vi "Sequence.Test.Load.Ready.vi"(9 "#products in the machine":i32, 10 "Data in":T9, 11 "Code in":T2={"Ready"=FALSE, "DoubleOrder"=FALSE, "OrderDone"=FALSE, "AllowSingleSlot"=FALSE, "CheckDM"=FALSE, "ThresholdA"=0, "ThresholdB"=0, "Plate"=enum."Wabco", "ImgPath"=path "", "Variant"={"State"=enum."Init", "ImgPath"=path "", "WabcoPlate"="", "WabcoProduct"="", "ClientProduct"="", "ClientPlate"="", "TotalQuantity"=0, "OrderQuantity"=0, "Serial"=0, "Wabco"={"LaserJob"="", "AdditionalTxt"="037", "FactoryCode"="", "RevID"=0, "ForkID"=0, "FailuresLimit"=0, "GlobalCnt"=0, "Bank"=0, "SerialFormat"=enum."6 dig", "CoordA"={"X"=0.0, "Y"=0.0, "Angle"=0.0}, "CoordB"={"X"=0.0, "Y"=0.0, "Angle"=0.0}, "DMCconfig"=0}, "Client"={"LaserJob"="", "AdditionalTxt"="", "FactoryCode"="037", "RevID"=0, "ForkID"=0, "FailuresLimit"=0, "GlobalCnt"=0, "Bank"=0, "SerialFormat"=enum."6 dig", "CoordA"={"X"=0.0, "Y"=0.0, "Angle"=0.0}, "CoordB"={"X"=0.0, "Y"=0.0, "Angle"=0.0}, "DMCconfig"=0}}}) -> (1 "Ready":bool, 2 "Loaded":bool, 3 "StatusFlags":T1)   [LabVIEW 2016]
uses:
  Sequence.Test.Status.ctl
  Sequence.Slot.StatusData.ctl
  Sequence.Test.Unload.Status.ctl
  Sequence.Prod.StatusData.ctl
  Sequence.Step.Status.ctl
  Sequence.Test.BreakReason.ctl
  Sequence.Code.Sets.ctl
  Sequence.PlateType.ctl
  Logger/Logger.Variant.Sets.ctl
  Station/Station.Changeover.State.vi
  Station/Station.Plate.Properties.ctl
  Sequence.Code.SerialFormat.ctl
  Drivers/V7310/LowLevel/V7310.Job.Sets.ctl
  Sequence.SerialsFglb.StatusFlags.ctl
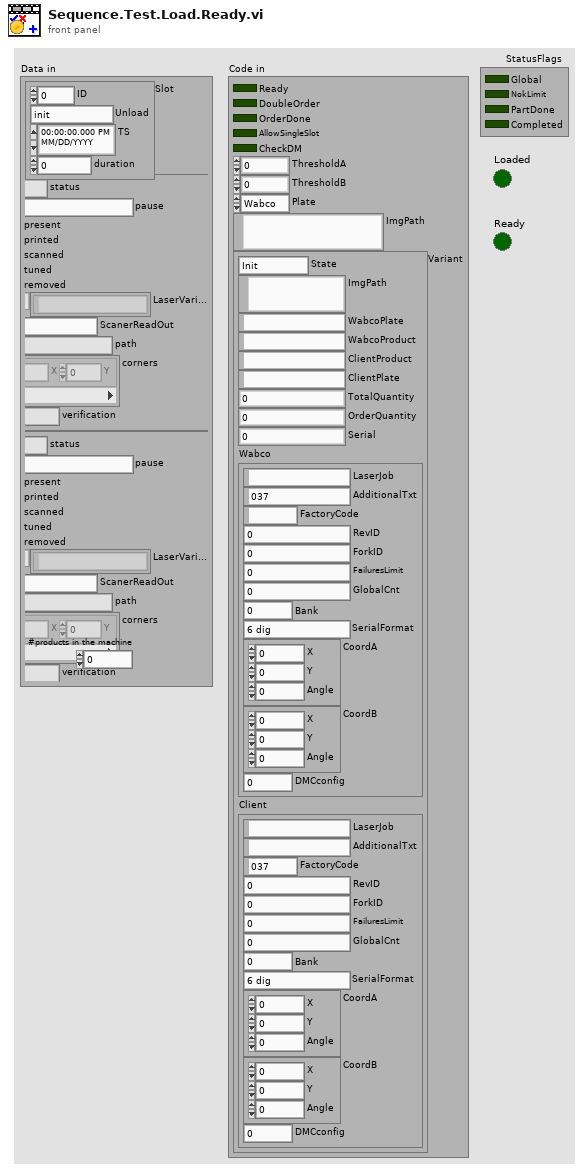
[diagram p1: front panel]
types:
  T1 = typedef "Sequence.SerialsFglb.StatusFlags.ctl" = cluster{"Global":bool, "NokLimit":bool, "PartDone":bool, "Completed":bool}
  T2 = typedef "Sequence.Code.Sets.ctl" = cluster{"Ready":bool, "DoubleOrder":bool, "OrderDone":bool, "AllowSingleSlot":bool, "CheckDM":bool, "ThresholdA":u8, "ThresholdB":u8, "Plate":T3, "ImgPath":path, "Variant":T4}
  T3 = typedef "Sequence.PlateType.ctl" = enum16{"Wabco", "Client"}
  T4 = typedef "Logger.Variant.Sets.ctl" = cluster{"State":T5, "ImgPath":path, "WabcoPlate":string, "WabcoProduct":string, "ClientProduct":string, "ClientPlate":string, "TotalQuantity":u16, "OrderQuantity":u16, "Serial":i32, "Wabco":T6, "Client":T6}
  T5 = typedef "Station.Changeover.State.vi" = enum16{"Init", "Scaning", "NOK", "Wait for ack", "Ready"}
  T6 = typedef "Station.Plate.Properties.ctl" = cluster{"LaserJob":string, "AdditionalTxt":string, "FactoryCode":string, "RevID":u8, "ForkID":u8, "FailuresLimit":u16, "GlobalCnt":i32, "Bank":u8, "SerialFormat":T7, "CoordA":T8, "CoordB":T8, "DMCconfig":i32}
  T7 = typedef "Sequence.Code.SerialFormat.ctl" = enum8{"", "6 dig", "7 dig"}
  T8 = typedef "V7310.Job.Sets.ctl" = cluster{"X":dbl, "Y":dbl, "Angle":dbl}
  T9 = typedef "Sequence.Test.Status.ctl" = cluster{"Slot":T10, "A":T12, "B":T12}
  T10 = typedef "Sequence.Slot.StatusData.ctl" = cluster{"ID":i32, "Unload":T11, "TS":timestamp, "duration":u32}
  T11 = typedef "Sequence.Test.Unload.Status.ctl" = enum16{"init", "check NOK", "check OK", "wait on NOK", "wait on OK", "wait on Unload", "done"}
  T12 = typedef "Sequence.Prod.StatusData.ctl" = cluster{"status":T13, "pause":T14, "present":bool, "printed":bool, "scanned":bool, "tuned":bool, "removed":bool, "LaserVariables":string[], "ScanerReadOut":string, "path":path, "corners":cluster{"X":i32, "Y":i32}[], "verification":u8}
  T13 = typedef "Sequence.Step.Status.ctl" = enum16{"-", "Pending", "Running", "Skipped", "Passed", "Failed", "Done", "Error", "Aborted", "Stopped"}
  T14 = typedef "Sequence.Test.BreakReason.ctl" = enum16{"-", "NOK container", "OK container", "Rev empty", "Rev missing", "Rev wrong", "Fork missing", "Fork wrong", "NOK limit", "Unload failure", "Single slot", "Part done", "Err: Prod move work", "Err: Prod move home", "Err: Prod lift work", "Err: Prod lift home", "Err: Prod Arm Work", "Err: Prod Arm NOK", "Err: Prod Arm OK", "Err: Prod NOK suck", "Err: Prod NOK drop", "Err: Prod OK missing", "Err: Prod OK suck", "Err: Prod OK drop"}
  T15 = typedef "Sequence.Counters.ctl" = cluster{"Expected":u16, "Done":u16, "OK":u16, "NOK":u16, "NOKlimit":u16, "Part":u16, "PartOK":u16}
  T16 = typedef "FestoCPX.Station.ProdPresent.ctl" = cluster{"Slot1":cluster{"A":bool, "B":bool}, "Slot2":cluster{"A":bool, "B":bool}, "Slot3":cluster{"A":bool, "B":bool}, "Slot4":cluster{"A":bool, "B":bool}, "Final":cluster{"A":bool, "B":bool}, "OK":cluster{"A":bool, "B":bool}, "Container":cluster{"OK":bool, "NOK":bool}}
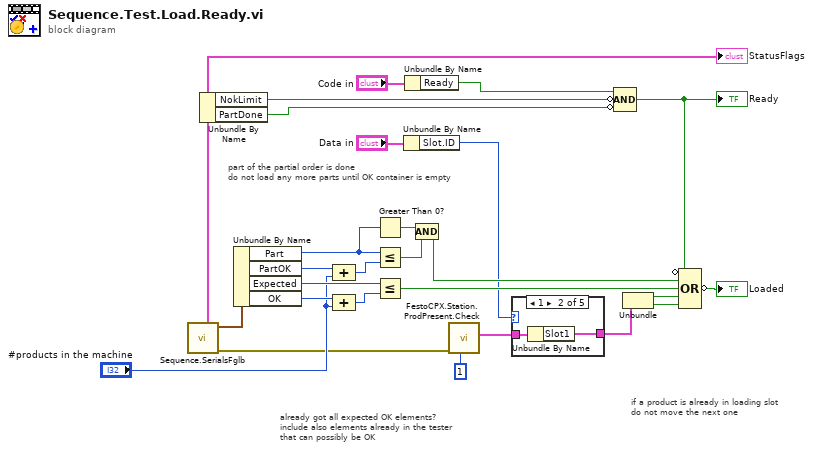
[diagram p0: block diagram]
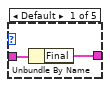
[diagram p2: hidden frame]
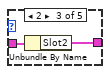
[diagram p3: hidden frame]
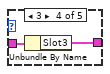
[diagram p4: hidden frame]
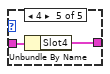
[diagram p5: hidden frame]
diagram:
  # "part of the partial order is done\ndo not load any more parts until OK container is empty"
  # "if a product is already in loading slot \ndo not move the next one"
  # "already got all expected OK elements?\ninclude also elements already in the tester\nthat can possibly be OK"
  n1 = call "Sequence.SerialsFglb.vi"() -> ("error out"=w4:errorcluster, "Counters out"=w11:T15, "StatusFlags"=w10:T1)  [unwired: 7 in, 2 out]
  "StatusFlags" <- w10
  n2 = Unbundle By Name(w10) -> ("NokLimit"=w12:bool, "PartDone"=w8:bool)
  n3 = Unbundle By Name(w11) -> ("Part"=w9:u16, "PartOK"=w15:u16, "Expected"=w27:u16, "OK"=w18:u16)
  n4 = Compound Arithmetic op=ADD(w15, "#products in the machine") -> (w13:i32)
  n5 = Compound Arithmetic op=ADD(w18, "#products in the machine") -> (w14:i32)
  n6 = Greater Than 0?(x=w9) -> (x > 0?=w7:bool)
  n7 = Less Or Equal?(x=w9, y=w13) -> (x <= y?=w17:bool)
  n8 = Less Or Equal?(x=w27, y=w14) -> (x <= y?=w26:bool)
  n9 = Unbundle By Name("Data in") -> ("Slot.ID"=w2:i32)
  n10 = Unbundle By Name("Code in") -> ("Ready"=w22:bool)
  n11 = Compound Arithmetic op=AND(w7, w17) -> (w16:bool)
  n12 = call "FestoCPX.Station.ProdPresent.Check.vi"("Stab Counter (0)"=1 ("Max Stab time [ms] (0)"), "error in"=w4) -> ("Prod Present"=w5:T16)  [unwired: 4 in, 5 out]
  n13 = case shown="1" w2 {
    tunnel: w5 -> [w29 w31 w33 w35 w37]
    tunnel: [w28 w30 w32 w34 w36] -> w3
    frame Default {
      n14 = Unbundle By Name(w29) -> ("Final"=w28:cluster{"A":bool, "B":bool})
    }
    frame 1 {
      n15 = Unbundle By Name(w31) -> ("Slot1"=w30:cluster{"A":bool, "B":bool})
    }
    frame 2 {
      n16 = Unbundle By Name(w33) -> ("Slot2"=w32:cluster{"A":bool, "B":bool})
    }
    frame 3 {
      n17 = Unbundle By Name(w35) -> ("Slot3"=w34:cluster{"A":bool, "B":bool})
    }
    frame 4 {
      n18 = Unbundle By Name(w37) -> ("Slot4"=w36:cluster{"A":bool, "B":bool})
    }
  }
  n19 = Compound Arithmetic op=AND(w22, invert w12, invert w8) -> (w20:bool)
  "Ready" <- w20
  n20 = Unbundle(w3) -> ("A"=w21:bool, "B"=w19:bool)
  n21 = Compound Arithmetic op=OR(invert w20, w16, w26, w21, w19) -> (invert →"Loaded":bool)
